vi "Configure Initiate Continuous.vi"(8 "error in (no error)":errorcluster {"code" format="%.0x"}, 10 "initiate continuous (True)":bool=TRUE caption="Initiate Continuous (True)", 11 "VISA Resource Name":refnum<visa-resource-name>) -> (0 "error out":errorcluster {"code" format="%.0x"}, 3 "VISA Resource Name Out":refnum<visa-resource-name>)   [LabVIEW 2011, in "Agilent 546XX Series.lvlib"]
doc: "This VI sets the continuous acquisition mode on the instrument."
uses:
  Agilent 546XX Series.lvlib
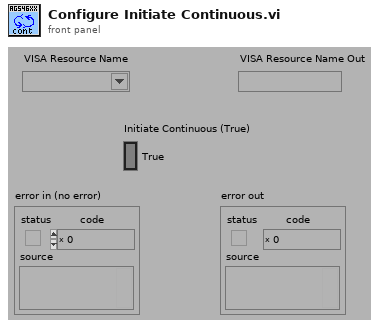
[diagram p1: front panel]
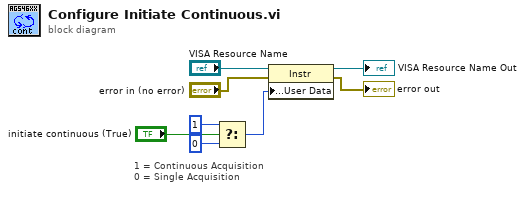
[diagram p0: block diagram]
diagram:
  # "1 = Continuous Acquisition\n0 = Single Acquisition"
  n1 = Select(t=u32 1, s="initiate continuous (True)", f=u32 0) -> (s? t:f=w3:u32)
  n2 = property class="Instr"(reference="VISA Resource Name", error in="error in (no error)", "General Settings:User Data"=w3) -> (reference out=→"VISA Resource Name Out":refnum<visa-resource-name>, error out=→"error out":errorcluster)
